vi "dynamixel_units_to_degrees.vi"(10 "MX Motor? (T)":bool=TRUE, 11 "Dynamixel Input":dbl) -> (2 "Dynamixel units/cycle":dbl, 3 "Degrees":dbl)   [LabVIEW 2013]
doc: "This VI takes in Dynamixel units and outputs degrees. The units are different for the MX and AX, which is controlled by the input boolean."
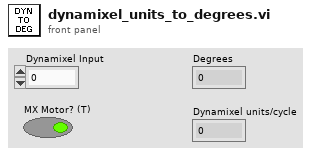
[diagram p1: front panel]
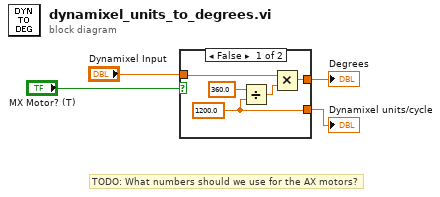
[diagram p0: block diagram]
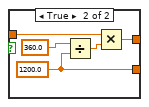
[diagram p2: hidden frame]
diagram:
  # "TODO: What numbers should we use for the AX motors?"
  n1 = case shown="False" "MX Motor? (T)" {
    tunnel: [w6 w10] -> w4
    tunnel: "Dynamixel Input" -> [w7 w14]
    tunnel: [w8 w13] -> w2
    frame False {
      w6 = 1200.0 ("y")
      n2 = Divide(x=360.0 ("y"), y=w6) -> (x/y=w9:dbl)
      n3 = Multiply(x=w7, y=w9) -> (x*y=w8:dbl)
    }
    frame True {
      w10 = 1200.0 ("y")
      n4 = Divide(x=360.0 ("y"), y=w10) -> (x/y=w12:dbl)
      n5 = Multiply(x=w14, y=w12) -> (x*y=w13:dbl)
    }
  }
  "Dynamixel units/cycle" <- w4
  "Degrees" <- w2
